vi "Korad_DC_supply_controller_BM.vi"(5 "COM Port":refnum<visa-resource-name>="COM9", 7 "Master Output Control":bool, 8 "Current":string="1.0", 9 "Voltage":string="4.0", 11 "Channel":string="1") -> ()   [LabVIEW 2021]
uses:
  <vilib>/Instr/_visa.llb/VISA Configure Serial Port (Instr).vi
panel:
  out "error out":errorcluster
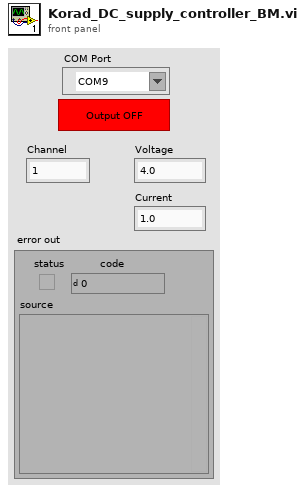
[diagram p1: front panel]
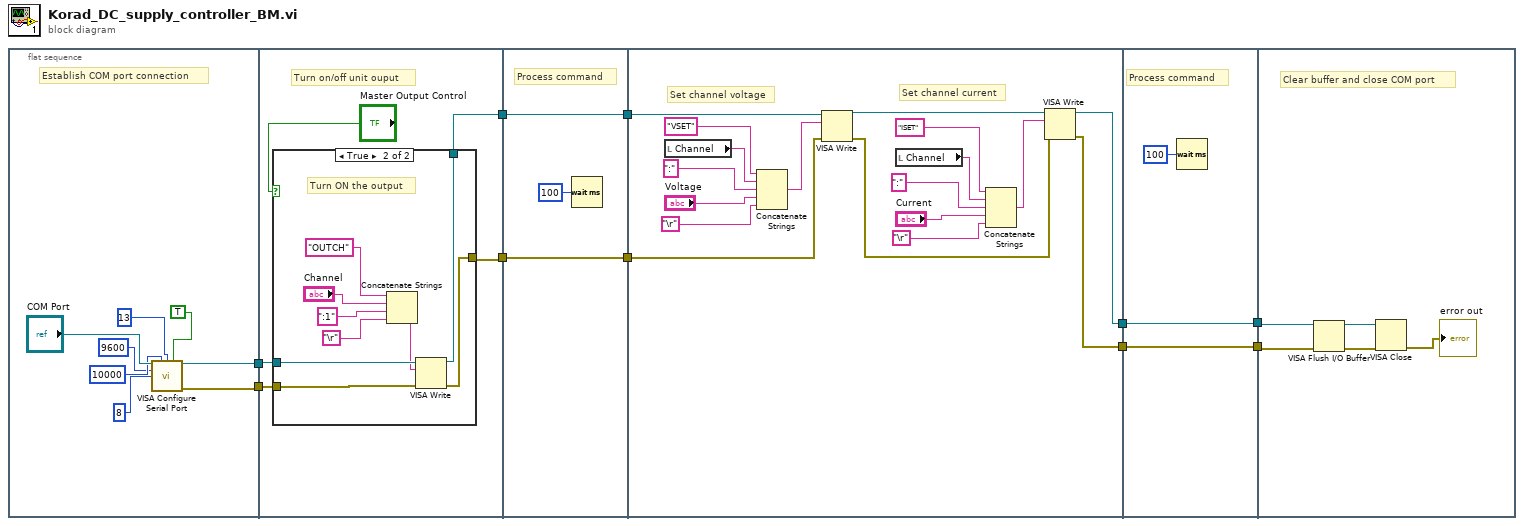
[diagram p0: block diagram]
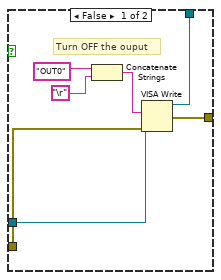
[diagram p2: hidden frame]
diagram:
  n1 = flat-sequence {
    tunnel: [w18] -> w3
    tunnel: [w17] -> w2
    tunnel: w3 -> [w19]
    tunnel: [w21] -> w10
    tunnel: w2 -> [w20]
    tunnel: [w22] -> w9
    tunnel: w10 -> [w42]
    tunnel: [w42] -> w5
    tunnel: w9 -> [w41]
    tunnel: [w41] -> w4
    tunnel: [w44] -> w8
    tunnel: w5 -> [w59]
    tunnel: w4 -> [w60]
    tunnel: [w43] -> w1
    tunnel: [w62] -> w7
    tunnel: [w61] -> w6
    tunnel: w8 -> [w61]
    tunnel: w1 -> [w62]
    tunnel: w7 -> [w66]
    tunnel: w6 -> [w65]
    frame #0 {
      # "Establish COM port connection"
      n2 = call-poly "VISA Configure Serial Port"("VISA resource name"="COM Port", "timeout (10sec)"=u32 10000, "termination char\n(0xA = '\\n' = LF)"=u8 13 ("termination char\n(0xA = '\\n' = LF)"), "Enable Termination\nChar (T)"=TRUE ("Enable Termination\nChar (T)"), "baud rate (9600)"=u32 9600, "data bits (8)"=u16 8) -> ("VISA resource name out"=w17:refnum<visa-resource-name>, "error out"=w18:errorcluster)  [unwired: 3 in, 5 out]
    }
    frame #1 {
      # "Turn on/off unit ouput"
      n3 = case shown="True" "Master Output Control" {
        tunnel: w20 -> [w30 w39]
        tunnel: w19 -> [w27 w38]
        tunnel: [w29 w37] -> w22
        tunnel: [w28 w36] -> w21
        frame False {
          # "Turn OFF the ouput"
          n4 = Concatenate Strings("OUT0" ("write buffer"), "\r") -> (w24:string)
          n5 = VISA Write(VISA resource name=w30, write buffer=w24, error in (no error)=w27) -> (VISA resource name out=w29:refnum<visa-resource-name>, error out=w28:errorcluster)  [unwired: 1 out]
        }
        frame True {
          # "Turn ON the output"
          n6 = Concatenate Strings("OUTCH" ("write buffer"), "Channel", ":1" ("string"), "\r") -> (w34:string)
          n7 = VISA Write(VISA resource name=w39, write buffer=w34, error in (no error)=w38) -> (VISA resource name out=w37:refnum<visa-resource-name>, error out=w36:errorcluster)  [unwired: 1 out]
        }
      }
    }
    frame #2 {
      # "Process command"
      n8 = Wait (ms)(milliseconds to wait=u32 100) -> ()  [unwired: 1 out]
    }
    frame #3 {
      # "Set channel current"
      # "Set channel voltage"
      n9 = local read "Channel"() -> (w49:string)
      n10 = Concatenate Strings("VSET" ("string"), w49, ":" ("string"), "Voltage", "\r") -> (w58:string)
      n11 = VISA Write(VISA resource name=w60, write buffer=w58, error in (no error)=w59) -> (VISA resource name out=w45:refnum<visa-resource-name>, error out=w46:errorcluster)  [unwired: 1 out]
      n12 = local read "Channel"() -> (w47:string)
      n13 = Concatenate Strings("ISET" ("string"), w47, ":" ("string"), "Current", "\r") -> (w53:string)
      n14 = VISA Write(VISA resource name=w45, write buffer=w53, error in (no error)=w46) -> (VISA resource name out=w43:refnum<visa-resource-name>, error out=w44:errorcluster)  [unwired: 1 out]
    }
    frame #4 {
      # "Process command"
      n15 = Wait (ms)(milliseconds to wait=u32 100) -> ()  [unwired: 1 out]
    }
    frame #5 {
      # "Clear buffer and close COM port"
      n16 = VISA Flush I/O Buffer(VISA resource name=w66, error in (no error)=w65) -> (VISA resource name out=w67:refnum<visa-resource-name>, error out=w64:errorcluster)  [unwired: 1 in]
      n17 = VISA Close(VISA resource name=w67, error in (no error)=w64) -> (error out=→"error out":errorcluster)
    }
  }
